vi "HAPS_LoadTable_SetBeam_Manual_TroubleShooting.vi"() -> ()   [LabVIEW 2023, in "HAPS.lvlib"]
uses:
  HAPS.lvlib
  HAPS_MCU_ELE_Func.ctl
  HAPS_SerialPort.ctl
  R_S/R_S.lvlib
  <vilib>/Utility/file.llb/Read Delimited Spreadsheet (string).vi
  set_ele.ctl
panel:
  in  "Simulation":bool=TRUE
  in  "OFF 13~15":bool
  in  "Init?":bool=TRUE
  in  "set_ele":T1={"ch"=0, "chain_id"=0, "group"=0, "array_id"=0, "ele_phase"=0, "ele_gain"=0, "com_gain"=17, "pd_range"=0}
  in  "file path (dialog if empty)":path=path "D:/_Project/_Code/LabVIEW/_CLC_Gen4/CLC_LV2023/CLC_Cali/Log/HAPS/Preset.csv"
  in  "VISA resource name":refnum<visa-resource-name>="COM1"
  out "Remaining quantity":i32
  out "ele phase":i32
  out "ele gain":i32
  out "channel":i32
  out "chain ID":i32
  out "group":i32
  out "array id":i32
  # "HAPS 24x24 Setting\nManual In-Phase_One"
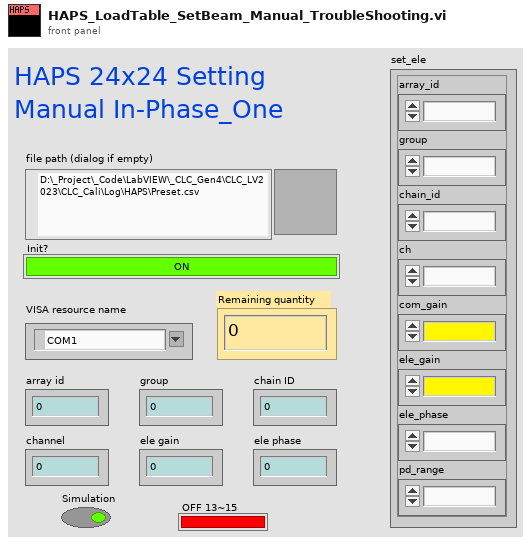
[diagram p1: front panel]
types:
  T1 = typedef "HAPS.lvlib/set_ele.ctl" = cluster{"ch":i32, "chain_id":i32, "group":i32, "array_id":i32, "ele_phase":i32, "ele_gain":i32, "com_gain":i32, "pd_range":i32}
  T2 = typedef "HAPS.lvlib/HAPS_SerialPort.ctl" = enum16{"Init", "Close", "CMD", "Flush"}
  T3 = typedef "HAPS.lvlib/HAPS_MCU_ELE_Func.ctl" = enum16{"array_init", "set_com_gain", "set_ch_gain_phase", "set_pd_range", "get_preamp_temp", "get_bfic_temp", "get_tx_pd", "ch_on", "ch_on_2", "ch_ctrl_all", "array_ctrl_src"}
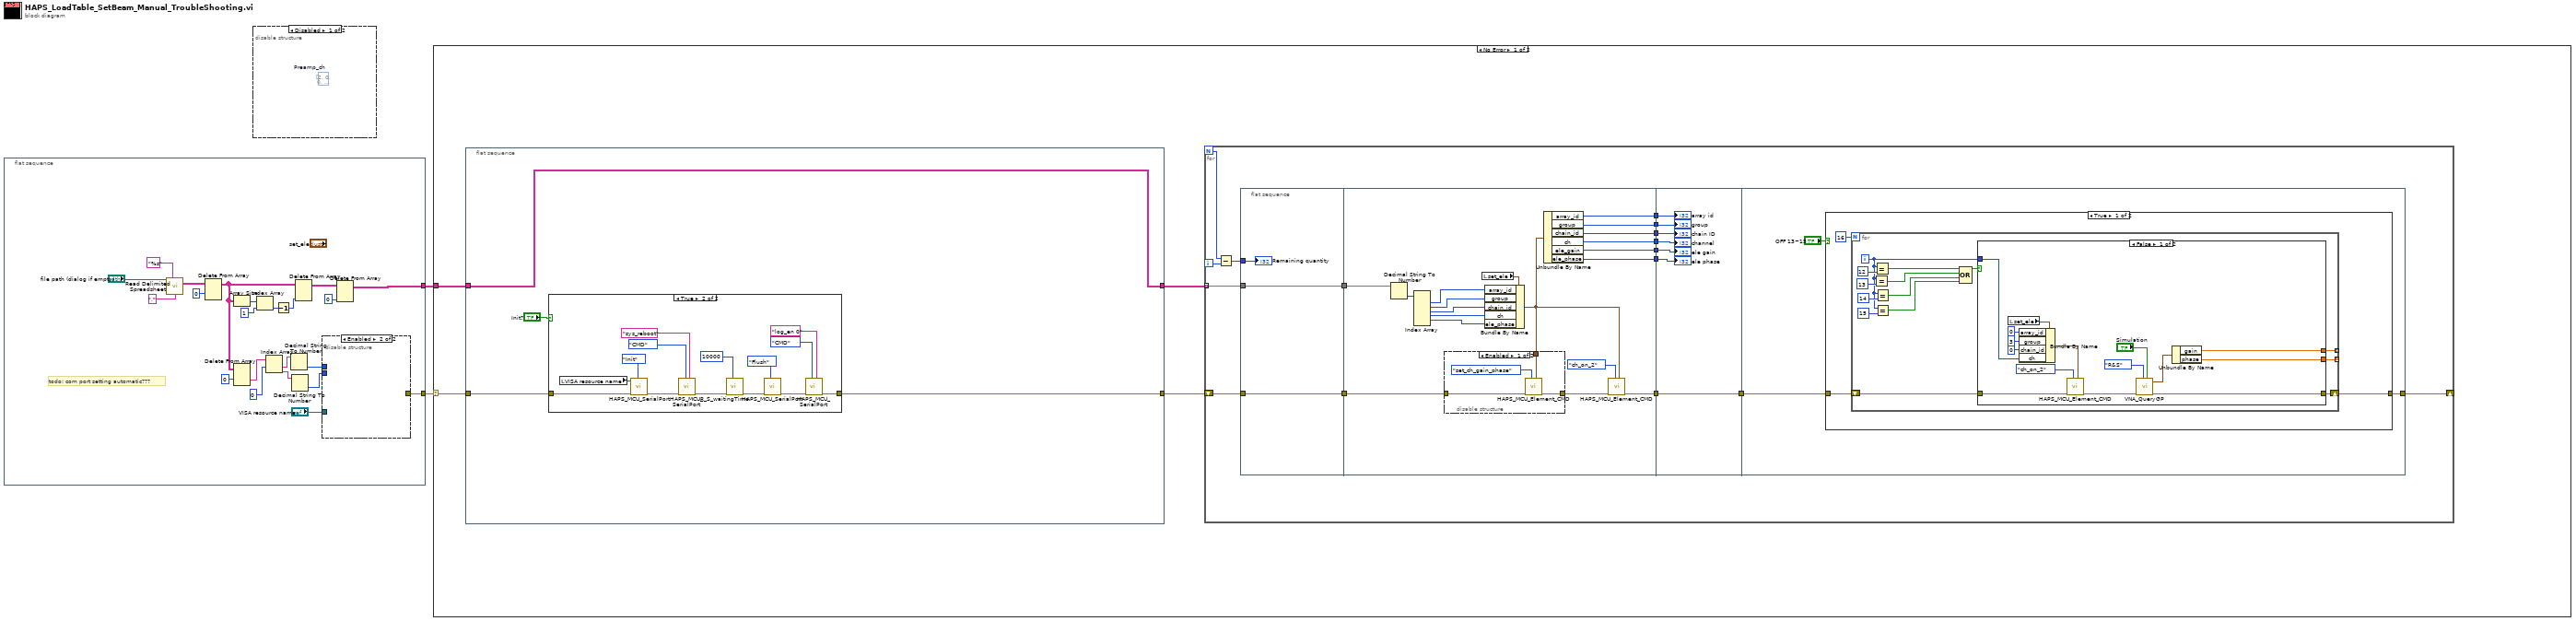
[diagram p0: block diagram]
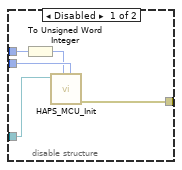
[diagram p2: hidden frame]
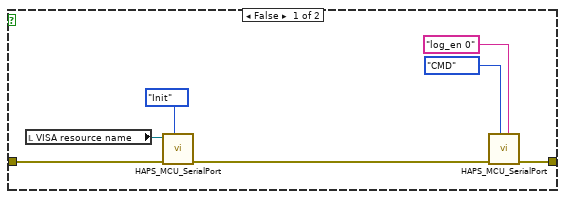
[diagram p4: hidden frame]
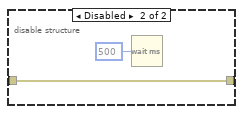
[diagram p5: hidden frame]
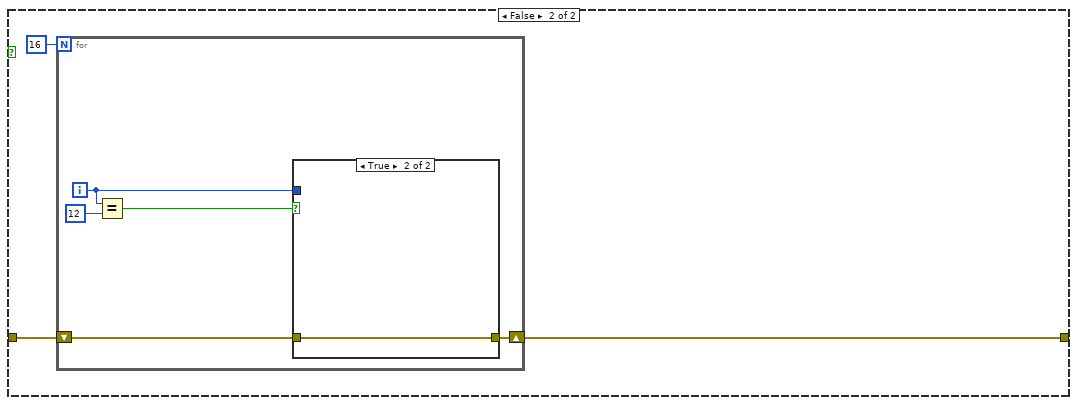
[diagram p7: hidden frame]
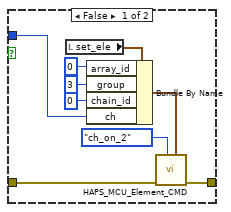
[diagram p8: hidden frame]
diagram:
  n1 = flat-sequence {
    tunnel: [w16] -> w2
    tunnel: [w3] -> w1
    frame #0 {
      # "todo: com port setting automatic???"
      n2 = call-poly <vilib>:"Read Delimited Spreadsheet.vi"("file path (dialog if empty)"="file path (dialog if empty)", "format (%s)"="%s" ("format (%.3f)"), "delimiter (\\t)"="," ("delimiter (\\t)")) -> ("all rows"=w22:string[][])  [unwired: 7 in, 5 out]
      n3 = Delete From Array(array=w22, index (row)=0) -> (array with subset deleted=w12:string[][])  [unwired: 2 in, 1 out]
      n4 = Array Size(array=w12) -> (size(s)=w20:i32[])
      n5 = Delete From Array(array=w12, index (row)=0) -> (deleted portion=w11:string[])  [unwired: 2 in, 1 out]
      n6 = Index Array(array=w20, index=1) -> (element=w17:i32)
      n7 = Index Array(array=w11, index #1=0 ("index")) -> (element #1=w10:string, element #2=w9:string)  [unwired: 1 in]
      n8 = Decrement(x=w17) -> (x-1=w19:i32)
      n9 = Decimal String To Number(string=w10) -> (number=w6:i32)  [unwired: 2 in, 1 out]
      n10 = Decimal String To Number(string=w9) -> (number=w5:i32)  [unwired: 2 in, 1 out]
      n11 = Delete From Array(array=w12, index (col)=w19) -> (array with subset deleted=w15:string[][])  [unwired: 2 in, 1 out]
      n12 = disable-structure shown="Enabled" {
        disable-tunnel: [w29 _] -> w16
        disable-tunnel: w6 -> [w28 _]
        disable-tunnel: w5 -> [w27 _]
        disable-tunnel: "VISA resource name" -> [w26 _]
        frame Disabled {
          n13 = To Unsigned Word Integer(number=w28) -> (unsigned 16bit integer=w25:u16)
          n14 = call "HAPS_MCU_Init.vi"("array_id"=w27, "Tx/Rx"=w25, "VISA resource name"=w26) -> ("error out"=w29:errorcluster)  [unwired: 8 in]
        }
        frame Enabled {
        }
      }
      n15 = Delete From Array(array=w15, index (col)=0 ("index (row)")) -> (array with subset deleted=w3:string[][])  [unwired: 2 in, 1 out]
    }
  }
  n16 = disable-structure shown="Disabled" {
    frame Disabled {
      (unwired) i32[][] [[2, 0, 0, 8, 8, 10, 11, 9, 9, 1, 1, 3], [3, 1, 1, 9, 9, 11, 13, 15, 15, 7, 7, 5], [5, 7, 7, 15, 15, 13, 14, 14, 6, 6, 4, 12]]  # Preamp_ch
    }
    frame Enabled {
    }
  }
  n17 = case shown="No Error" w2 {
    selector: w2 -> [w31 _]
    tunnel: w1 -> [w33 _]
    frame No Error {
      n18 = flat-sequence {
        tunnel: w33 -> [w37]
        tunnel: [w37] -> w32
        tunnel: w31 -> [w36]
        tunnel: [w34] -> w30
        frame #0 {
          n19 = case shown="True" "Init?" {
            tunnel: w36 -> [w42 w56]
            tunnel: [w40 w54] -> w34
            frame False {
              n20 = local read "VISA resource name"() -> (w38:refnum<visa-resource-name>)
              n21 = call "HAPS_MCU_SerialPort.vi"("HAPS_SerialPort_Func"=HAPS_SerialPort."Init", "error in"=w42, "VISA resource name"=w38) -> ("error out"=w39:errorcluster)  [unwired: 6 in, 2 out]
              n22 = call "HAPS_MCU_SerialPort.vi"("Command"="log_en 0", "HAPS_SerialPort_Func"=enum16{"Init", "Close", "CMD"}."CMD" ("HAPS_SerialPort"), "error in"=w39) -> ("error out"=w40:errorcluster)  [unwired: 6 in, 2 out]
            }
            frame True {
              n23 = local read "VISA resource name"() -> (w45:refnum<visa-resource-name>)
              n24 = call "HAPS_MCU_SerialPort.vi"("HAPS_SerialPort_Func"=HAPS_SerialPort."Init", "error in"=w56, "VISA resource name"=w45) -> ("error out"=w51:errorcluster)  [unwired: 6 in, 2 out]
              n25 = call "HAPS_MCU_SerialPort.vi"("Command"="sys_reboot", "HAPS_SerialPort_Func"=enum16{"Init", "Close", "CMD"}."CMD" ("HAPS_SerialPort"), "error in"=w51) -> ("error out"=w50:errorcluster)  [unwired: 6 in, 2 out]
              n26 = call "R_S_waitingTime.vi"("Waiting Time(ms)"=u32 10000, "error in"=w50) -> ("error out"=w48:errorcluster)  [unwired: 9 in]
              n27 = call "HAPS_MCU_SerialPort.vi"("HAPS_SerialPort_Func"=HAPS_SerialPort."Flush", "error in"=w48) -> ("error out"=w46:errorcluster)  [unwired: 7 in, 2 out]
              n28 = call "HAPS_MCU_SerialPort.vi"("Command"="log_en 0", "HAPS_SerialPort_Func"=enum16{"Init", "Close", "CMD"}."CMD" ("HAPS_SerialPort"), "error in"=w46) -> ("error out"=w54:errorcluster)  [unwired: 6 in, 2 out]
            }
          }
        }
      }
      n29 = for {
        N -> [w68]
        tunnel: w32 -> [w74] mode=indexing
        shift-right: [w73] -> _
        shift-left: w30 -> [w72]
        i -> [w69]
        n30 = Subtract(x=w68, y=w69) -> (x-y=w67:i32)
        n31 = flat-sequence {
          tunnel: w72 -> [w77]
          tunnel: w74 -> [w75]
          tunnel: [w75] -> w71
          tunnel: [w77] -> w70
          tunnel: w67 -> [w76]
          tunnel: w71 -> [w96]
          tunnel: w70 -> [w94]
          tunnel: [w81] -> w66
          tunnel: [w90] -> w65
          tunnel: [w89] -> w64
          tunnel: [w88] -> w63
          tunnel: [w87] -> w62
          tunnel: [w86] -> w61
          tunnel: [w85] -> w60
          tunnel: w66 -> [w109]
          tunnel: w65 -> [w108]
          tunnel: w64 -> [w107]
          tunnel: w63 -> [w106]
          tunnel: w62 -> [w105]
          tunnel: w61 -> [w104]
          tunnel: w60 -> [w103]
          tunnel: [w109] -> w59
          tunnel: [w110] -> w73
          tunnel: w59 -> [w111]
          frame #0 {
            "Remaining quantity" <- w76
          }
          frame #1 {
            n32 = Decimal String To Number(string=w96) -> (number=w95:i32[])  [unwired: 2 in, 1 out]
            n33 = Index Array(array=w95) -> (element #1=w93:i32, element #2=w84:i32, element #3=w83:i32, element #4=w92:i32, element #5=w91:i32)  [unwired: 6 in, 1 out]
            n34 = local read "set_ele"() -> (w78:T1)
            n35 = Bundle By Name(cluster=w78, "array_id"=w93, "group"=w84, "chain_id"=w83, "ch"=w92, "ele_phase"=w91) -> (w79:T1)
            n36 = disable-structure shown="Enabled" {
              disable-tunnel: [w100 w102] -> w82
              disable-tunnel: w94 -> [w99 w102]
              disable-tunnel: w79 -> [w97 _]
              frame Enabled {
                n37 = call "HAPS_MCU_Element_CMD.vi"("set_ele"=w97, "HAPS_MCU_ELE_Func."=HAPS_MCU_ELE_Func."set_ch_gain_phase", "error in"=w99) -> ("error out"=w100:errorcluster)  [unwired: 7 in, 1 out]
              }
              frame Disabled {
                n38 = Wait (ms)(milliseconds to wait=u32 500) -> ()  [unwired: 1 out]
              }
            }
            n39 = Unbundle By Name(w79) -> ("array_id"=w90:i32, "group"=w89:i32, "chain_id"=w88:i32, "ch"=w87:i32, "ele_gain"=w86:i32, "ele_phase"=w85:i32)
            n40 = call "HAPS_MCU_Element_CMD.vi"("set_ele"=w79, "HAPS_MCU_ELE_Func."=HAPS_MCU_ELE_Func."ch_on_2", "error in"=w82) -> ("error out"=w81:errorcluster)  [unwired: 7 in, 1 out]
          }
          frame #2 {
            "group" <- w107
            "chain ID" <- w106
            "channel" <- w105
            "ele gain" <- w104
            "ele phase" <- w103
            "array id" <- w108
          }
          frame #3 {
            n41 = case shown="True" "OFF 13~15" {
              tunnel: [w114 w147] -> w110
              tunnel: w111 -> [w113 w146]
              frame True {
                n42 = for {
                  N: 16 -> [_]
                  shift-right: [w128] -> w114
                  shift-left: w113 -> [w129]
                  tunnel: [w117] -> _ mode=indexing
                  tunnel: [w116] -> _ mode=indexing
                  i -> [w119]
                  n43 = Equal?(x=w119, y=13) -> (x = y?=w123:bool)
                  n44 = Equal?(x=w119, y=12) -> (x = y?=w127:bool)
                  n45 = Equal?(x=w119, y=14) -> (x = y?=w121:bool)
                  n46 = Equal?(x=w119, y=15) -> (x = y?=w118:bool)
                  n47 = Compound Arithmetic op=OR(w127, w123, w121, w118) -> (w124:bool)
                  n48 = case shown="False" w124 {
                    tunnel: w129 -> [w138 w145]
                    tunnel: [w135 w145] -> w128
                    tunnel: w119 -> [w137 _]
                    tunnel: [w131 _] -> w116
                    tunnel: [w130 _] -> w117
                    frame False {
                      n49 = local read "set_ele"() -> (w140:T1)
                      n50 = Bundle By Name(cluster=w140, "array_id"=0, "group"=3, "chain_id"=0, "ch"=w137) -> (w141:T1)
                      n51 = call "HAPS_MCU_Element_CMD.vi"("set_ele"=w141, "HAPS_MCU_ELE_Func."=HAPS_MCU_ELE_Func."ch_on_2", "error in"=w138) -> ("error out"=w136:errorcluster)  [unwired: 7 in, 1 out]
                      n52 = call "VNA_QueryGP.vi"("Simulation"="Simulation", "HAPS_Equipment"=enum16{"Keysight", "R&S"}."R&S", "error in"=w136) -> ("error out"=w135:errorcluster, "queryMarker"=w132:cluster{"gain":dbl, "phase":dbl})  [unwired: 7 in]
                      n53 = Unbundle By Name(w132) -> ("gain"=w131:dbl, "phase"=w130:dbl)
                    }
                    frame True {
                    }
                  }
                }
              }
              frame False {
                n54 = for {
                  N: 16 -> [_]
                  shift-right: [w152] -> w147
                  shift-left: w146 -> [w153]
                  i -> [w150]
                  n55 = Equal?(x=w150, y=12) -> (x = y?=w149:bool)
                  n56 = case shown="True" w149 {
                    tunnel: w153 -> [w156 w163]
                    tunnel: [w155 w163] -> w152
                    tunnel: w150 -> [w154 _]
                    frame False {
                      n57 = local read "set_ele"() -> (w158:T1)
                      n58 = Bundle By Name(cluster=w158, "array_id"=0, "group"=3, "chain_id"=0, "ch"=w154) -> (w159:T1)
                      n59 = call "HAPS_MCU_Element_CMD.vi"("set_ele"=w159, "HAPS_MCU_ELE_Func."=HAPS_MCU_ELE_Func."ch_on_2", "error in"=w156) -> ("error out"=w155:errorcluster)  [unwired: 7 in, 1 out]
                    }
                    frame True {
                    }
                  }
                }
              }
            }
          }
        }
      }
    }
    frame Error {
    }
  }
